vi "Read FPGA.vi"() -> (4 "Data":T1)   [LabVIEW 2019]
uses:
  Data.ctl
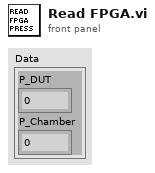
[diagram p1: front panel]
types:
  T1 = typedef "Data.ctl" = cluster{"P_DUT":dbl, "P_Chamber":dbl}
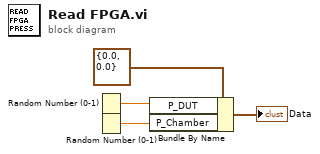
[diagram p0: block diagram]
diagram:
  n1 = Random Number (0-1)() -> (number: 0 to 1=w3:dbl)
  n2 = Random Number (0-1)() -> (number: 0 to 1=w4:dbl)
  n3 = Bundle By Name(cluster=T1 {"P_DUT"=0.0, "P_Chamber"=0.0} ("Data"), "P_DUT"=w3, "P_Chamber"=w4) -> (→"Data":T1)
